vi "Update Status Text.vi"(8 "error in (no error)":errorcluster, 11 "Response in":refnum<class "Response.lvclass">) -> (0 "error out":errorcluster, 3 "Response out":refnum<class "Response.lvclass">)   [LabVIEW 2020, in "HTTP Utils.lvlib" / "Response.lvclass"]
uses:
  Response.lvclass
  Response.lvclass/Response.ctl
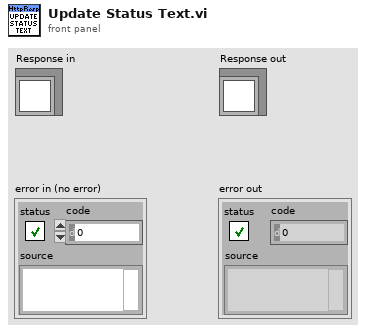
[diagram p1: front panel]
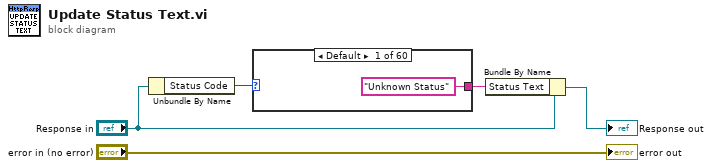
[diagram p0: block diagram]
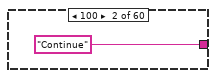
[diagram p2: hidden frame]
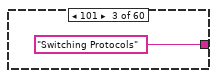
[diagram p3: hidden frame]
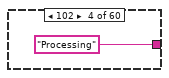
[diagram p4: hidden frame]
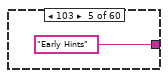
[diagram p5: hidden frame]
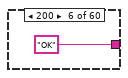
[diagram p6: hidden frame]
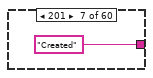
[diagram p7: hidden frame]
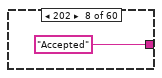
[diagram p8: hidden frame]
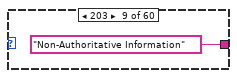
[diagram p9: hidden frame]
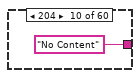
[diagram p10: hidden frame]
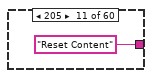
[diagram p11: hidden frame]
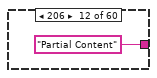
[diagram p12: hidden frame]
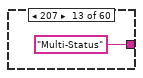
[diagram p13: hidden frame]
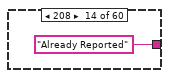
[diagram p14: hidden frame]
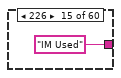
[diagram p15: hidden frame]
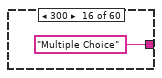
[diagram p16: hidden frame]
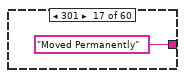
[diagram p17: hidden frame]
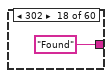
[diagram p18: hidden frame]
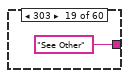
[diagram p19: hidden frame]
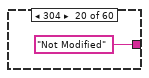
[diagram p20: hidden frame]
diagram:
  n1 = Unbundle By Name("Response in") -> ("Status Code"=w3:u16)
  n2 = case shown="Default" w3 {
    tunnel: ["Unknown Status" "Continue" "Switching Protocols" "Processing" "Early Hints" "OK" "Created" "Accepted" "Non-Authoritative Information" "No Content" "Reset Content" "Partial Content" "Multi-Status" "Already Reported" "IM Used" "Multiple Choice" "Moved Permanently" "Found" "See Other" "Not Modified" "Temporary Redirect" "Permanent Redirect" "Bad Request" "Unauthorized" "Forbidden" "404" "Method Not Allowed" "Not Acceptable" "Proxy Authentication Required" "Request Timeout" "Conflict" "Gone" "Length Required" "Precondition Failed" "Payload Too Large" "URI Too Long" "Unsupported Media Type" "Range Not Satisfiable" "Expectation Failed" "I'm a teapot" "Misdirected Request" "Unprocessable Entity" "Locked" "Failed Dependency" "Upgrade Required" "Precondition Required" "Too Many Requests" "Request Header Fields Too Large" "Unavailable For Legal Reasons" "Internal Server Error" "Not Implemented" "Bad Gateway" "Service Unavailable" "Gateway Timeout" "HTTP Version Not Supported" "Variant Also Negotiates" "Insufficient Storage" "Loop Detected" "Not Extended" "Network Authentication Required"] -> w1
    frame Default {
    }
    frame 100 {
    }
    frame 101 {
    }
    frame 102 {
    }
    frame 103 {
    }
    frame 200 {
    }
    frame 201 {
    }
    frame 202 {
    }
    frame 203 {
    }
    frame 204 {
    }
    frame 205 {
    }
    frame 206 {
    }
    frame 207 {
    }
    frame 208 {
    }
    frame 226 {
    }
    frame 300 {
    }
    frame 301 {
    }
    frame 302 {
    }
    frame 303 {
    }
    frame 304 {
    }
    frame 307 {
    }
    frame 308 {
    }
    frame 400 {
    }
    frame 401 {
    }
    frame 403 {
    }
    frame 404 {
    }
    frame 405 {
    }
    frame 406 {
    }
    frame 407 {
    }
    frame 408 {
    }
    frame 409 {
    }
    frame 410 {
    }
    frame 411 {
    }
    frame 412 {
    }
    frame 413 {
    }
    frame 414 {
    }
    frame 415 {
    }
    frame 416 {
    }
    frame 417 {
    }
    frame 418 {
    }
    frame 421 {
    }
    frame 422 {
    }
    frame 423 {
    }
    frame 424 {
    }
    frame 426 {
    }
    frame 428 {
    }
    frame 429 {
    }
    frame 431 {
    }
    frame 451 {
    }
    frame 500 {
    }
    frame 501 {
    }
    frame 502 {
    }
    frame 503 {
    }
    frame 504 {
    }
    frame 505 {
    }
    frame 506 {
    }
    frame 507 {
    }
    frame 508 {
    }
    frame 510 {
    }
    frame 511 {
    }
  }
  n3 = Bundle By Name(cluster="Response in", "Status Text"=w1) -> (→"Response out":refnum<class "Response.lvclass">)
  "error out" <- "error in (no error)"
